vi "1 Encoder PositionVelocity.vi"(0 "Encoder Input":refnum<k21>="Chassis1/Mod4/DI4", 2 "Encoder Interval (uSec)":u32=1000, 4 "Position Reset":bool) -> (7 "Encoder Packets":u64[](array[numeric]))   [LabVIEW 2010]
uses:
  <vilib>/eio/EIONode/EIONode.xnode
  <vilib>/rvi/eio/nirviEIOImplementation/nirviEIOImplementation.xnode
  <vilib>/rvi/eio/common/nirviEmuClasses.ctl
  <vilib>/rvi/eio/common/nirviEmuTemplateMethod_noerrors.vi
panel:
  out "Velocity (Counts/Interval)":i32
  out "Acceleration (Counts/Interval)":i32
  out "Position (Counts)":i32
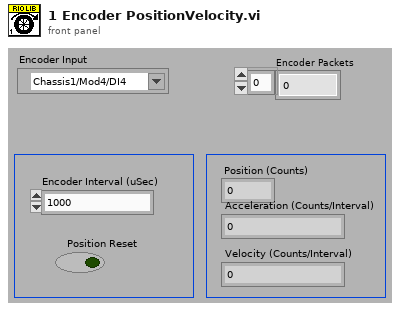
[diagram p1: front panel]
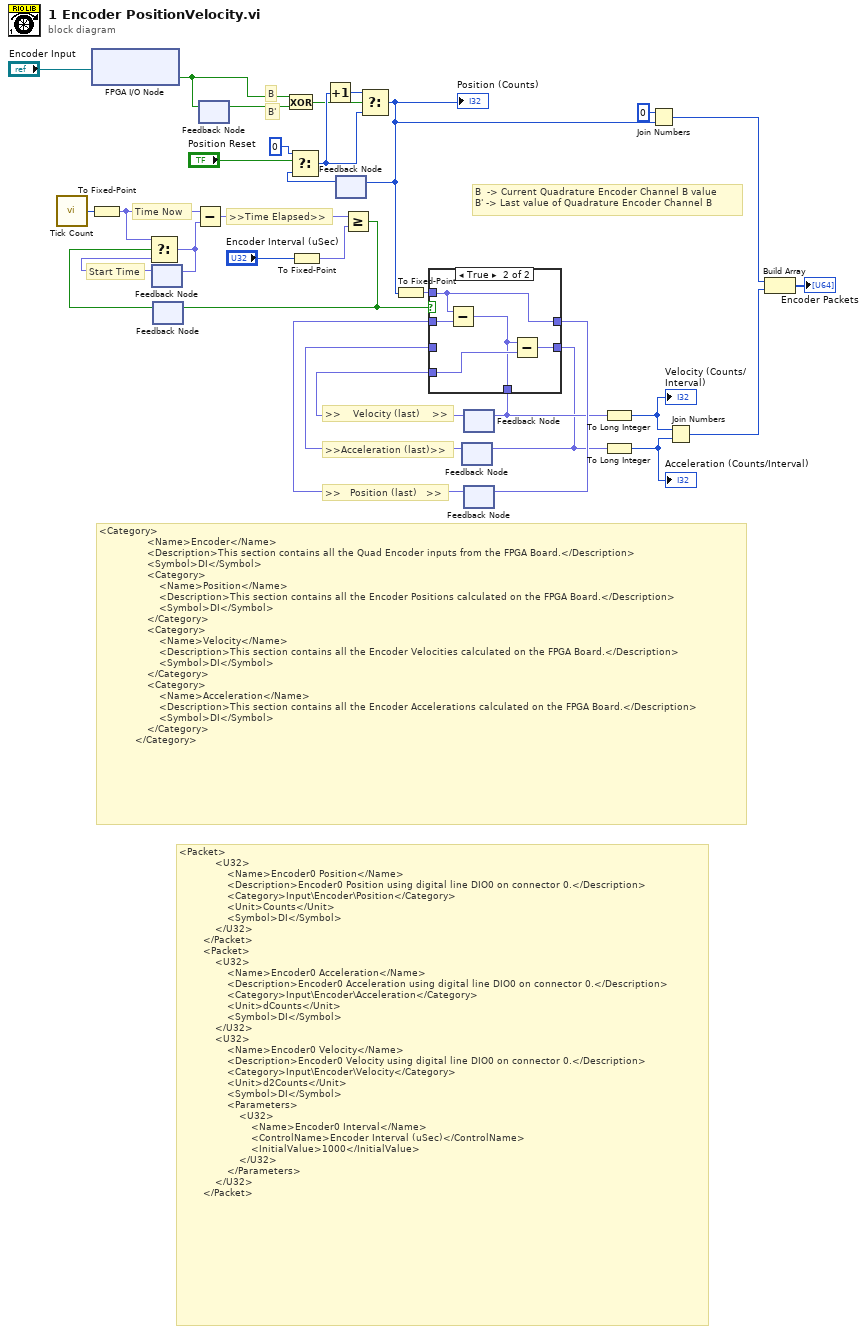
[diagram p0: block diagram]
diagram:
  # "<Category>\n                <Name>Encoder</Name>\n                <Description>This section contains all the Quad Encoder inputs from the FPGA Board.</Description>\n                <Symbol>DI</Symbol>\n                <Category>\n                    <Name>Position</Name>\n                    <Description>This section contains all the Encoder Positions calculated on the FPGA Board.</Description>\n                    <Symbol>DI</Symbol>\n                </Category>\n                <Category>\n                    <Name>Velocity</Name>\n                    <Description>This section contains all the Encoder Velocities calculated on the FPGA Board.</Description>\n                    <Symbol>DI</Symbol>\n                </Category>\n                <Category>\n                    <Name>Acceleration</Name>\n                    <Description>This section contains all the Encoder Accelerations calculated on the FPGA Board.</Description>\n                    <Symbol>DI</Symbol>\n                </Category>\n            </Category>"
  # "<Packet>\n            <U32>\n                <Name>Encoder0 Position</Name>\n                <Description>Encoder0 Position using digital line DIO0 on connector 0.</Description>\n                <Category>Input\\Encoder\\Position</Category>\n                <Unit>Counts</Unit>\n                <Symbol>DI</Symbol>\n            </U32>\n        </Packet>\n        <Packet>\n            <U32>\n                <Name>Encoder0 Acceleration</Name>\n                <Description>Encoder0 Acceleration using digital line DIO0 on connector 0.</Description>\n                <Category>Input\\Encoder\\Acceleration</Category>\n                <Unit>dCounts</Unit>\n                <Symbol>DI</Symbol>\n            </U32>\n            <U32>\n                <Name>Encoder0 Velocity</Name>\n                <Description>Encoder0 Velocity using digital line DIO0 on connector 0.</Description>\n                <Category>Input\\Encoder\\Velocity</Category>\n                <Unit>d2Counts</Unit>\n                <Symbol>DI</Symbol>\n                <Parameters>\n                    <U32>\n                        <Name>Encoder0 Interval</Name>\n                        <ControlName>Encoder Interval (uSec)</ControlName>\n                        <InitialValue>1000</InitialValue>\n                    </U32>\n                </Parameters>\n            </U32>\n        </Packet>"
  # "B  -> Current Quadrature Encoder Channel B value\nB' -> Last value of Quadrature Encoder Channel B"
  # ">>Acceleration (last)>>"
  # "Start Time"
  # "B'"
  # "B"
  # ">>    Velocity (last)    >>"
  # ">>   Position (last)   >>"
  # "Time Now"
  # ">>Time Elapsed>>"
  n1 = call "Tick Count"() -> ("Tick Count(uSec)"=w17:u32)
  n2 = xnode "FPGA I/O Node"("FPGA I/O In"="Encoder Input") -> ("I/O Item"=w19:bool)  [unwired: 1 out]
  n3 = To Fixed-Point(number=w17) -> (fixed-point=w5:fxp<+,32,32>)  [unwired: 1 in]
  n4 = feedback #1() -> (w25:fxp<+,32,32>)  [unwired: 1 in]
  n5 = feedback #2() -> (w27:bool)  [unwired: 1 in]
  n6 = Select(t=w5, s=w27, f=w25) -> (s? t:f=w6:fxp<+,32,32>)
  n7 = feedback-in #1(w6) -> ()
  n8 = Subtract(x=w5, y=w6) -> (x-y=w4:fxp<+,32,32>)
  n9 = feedback-in #3(w19) -> ()
  n10 = feedback #3() -> (w18:bool)  [unwired: 1 in]
  n11 = Exclusive Or(1:w18, 2:w19) -> (0:w9:bool)
  n12 = To Fixed-Point(number="Encoder Interval (uSec)") -> (fixed-point=w3:fxp<+,32,32>)  [unwired: 1 in]
  n13 = feedback #4() -> (w28:i32)  [unwired: 1 in]
  n14 = Select(t=0 ("32 bit"), s="Position Reset", f=w28) -> (s? t:f=w30:i32)
  n15 = Increment(x=w30) -> (x+1=w32:i32)
  n16 = Greater Or Equal?(x=w4, y=w3) -> (x >= y?=w24:bool)
  n17 = feedback-in #2(w24) -> ()
  n18 = Select(t=w32, s=w9, f=w30) -> (s? t:f=w16:i32)
  "Position (Counts)" <- w16
  n19 = feedback-in #4(w16) -> ()
  n20 = To Fixed-Point(number=w16) -> (fixed-point=w7:fxp<+/-,32,32>)  [unwired: 1 in]
  n21 = feedback #5() -> (w21:fxp<+/-,32,32>)  [unwired: 1 in]
  n22 = feedback #6() -> (w22:fxp<+/-,32,32>)  [unwired: 1 in]
  n23 = feedback #7() -> (w23:fxp<+/-,32,32>)  [unwired: 1 in]
  n24 = case shown="True" w24 {
    tunnel: w7 -> [_ w39]
    tunnel: w23 -> [w33 w40]
    tunnel: [w35 w37] -> w14
    tunnel: w22 -> [w35 w38]
    tunnel: [w34 w36] -> w13
    tunnel: w21 -> [w34 _]
    tunnel: [w33 w39] -> w20
    frame False {
    }
    frame True {
      n25 = Subtract(x=w39, y=w40) -> (x-y=w37:fxp<+/-,32,32>)
      n26 = Subtract(x=w37, y=w38) -> (x-y=w36:fxp<+/-,32,32>)
    }
  }
  n27 = feedback-in #5(w13) -> ()
  n28 = feedback-in #6(w14) -> ()
  n29 = feedback-in #7(w20) -> ()
  n30 = To Long Integer(number=w14) -> (32bit integer=w2:i32)
  "Velocity (Counts/Interval)" <- w2
  n31 = To Long Integer(number=w13) -> (32bit integer=w1:i32)
  "Acceleration (Counts/Interval)" <- w1
  n32 = Join Numbers(hi=0, lo=w16) -> ((hi.lo)=w12:u64)
  n33 = Join Numbers(hi=w2, lo=w1) -> ((hi.lo)=w11:u64)
  n34 = Build Array(w12, w11) -> (→"Encoder Packets":u64[])
